vi "机械手工具坐标转世界坐标.vi"(9 "最终的世界坐标角度(单位角度)":dbl=89.996 format="%#_13g", 11 "P-XYZR":T2) -> (1 "计算出来 世界坐标系坐标XYZR out":T2, 3 "计算出来 世界坐标系坐标 out":T1 {"X" format="%#.3f"})   [LabVIEW 2014]
uses:
  Controls/XYPos.ctl
  Controls/XYZRPos.ctl
  Global.vi
panel:
  in  "选项卡控件":enum32{"选项卡 1", "选项卡 2"}(tab)=enum."选项卡 2"
  in  "世界坐标 O点(旧 R=0)":T1={"X"=309.781, "Y"=-196.165} {"X" format="%#.3f"}
  in  "OK工具坐标(robot显示)":T1={"X"=310.034, "Y"=-196.847} {"X" format="%#.3f"}
  out "OK offset":T1 {"X" format="%#.3f"}
  out "算出来 M在旧坐标系坐标":T1 {"X" format="%#.3f"}
  out "坐标平移量":cluster{dbl, dbl}
  in  "OK工具坐标 2":T1={"X"=309.781, "Y"=-194.165} {"X" format="%#.3f"}
  out "OK offset 2":T1 {"X" format="%#.3f"}
  out "算出来 M在旧坐标系坐标 2":T1 {"X" format="%#.3f"}
  out "计算的-坐标平移量 2":cluster{dbl, dbl}
  out "算出来 M在旧坐标系坐标 3":T1 {"X" format="%#.3f"}
  out "OK offset 3":T1 {"X" format="%#.3f"}
  in  "OK工具坐标(robot显示) 2":T1={"X"=310.033, "Y"=-196.846} {"X" format="%#.3f"}
  in  "工具/世界坐标XY in":T1={"X"=310.033, "Y"=-196.846} {"X" format="%#.3f"}
  in  "H0角度(单位角度)":dbl format="%#_13g"
  out "计算的-坐标平移量 3":cluster{dbl, dbl}
  in  "H0半径":dbl format="%#_13g"
  # "90"
  # "10"
  # "对位后世界坐标为XY  R\n求旋转后世界坐标\n1. XYR 转换为工具坐标 X1 Y1  R  (注意：这里仍然用世界坐标角度)\n2  H0旋转30度，则X1 Y1 (R+30)  \n3， 则X1 Y1 (R+30)  转换成世界坐标"
  # "309.352"
  # "-197.099"
  # "注意：这里输入的是最终世界坐标角度"
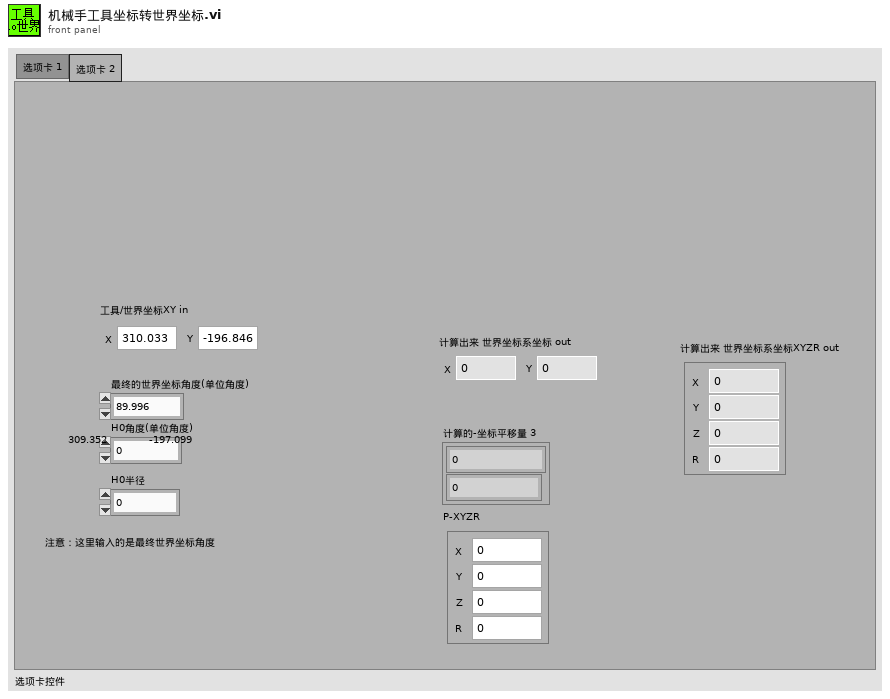
[diagram p1: front panel]
types:
  T1 = typedef "XYPos.ctl" = cluster{"X":dbl, "Y":dbl}
  T2 = typedef "XYZRPos.ctl" = cluster{"X":dbl, "Y":dbl, "Z":dbl, "R":dbl}
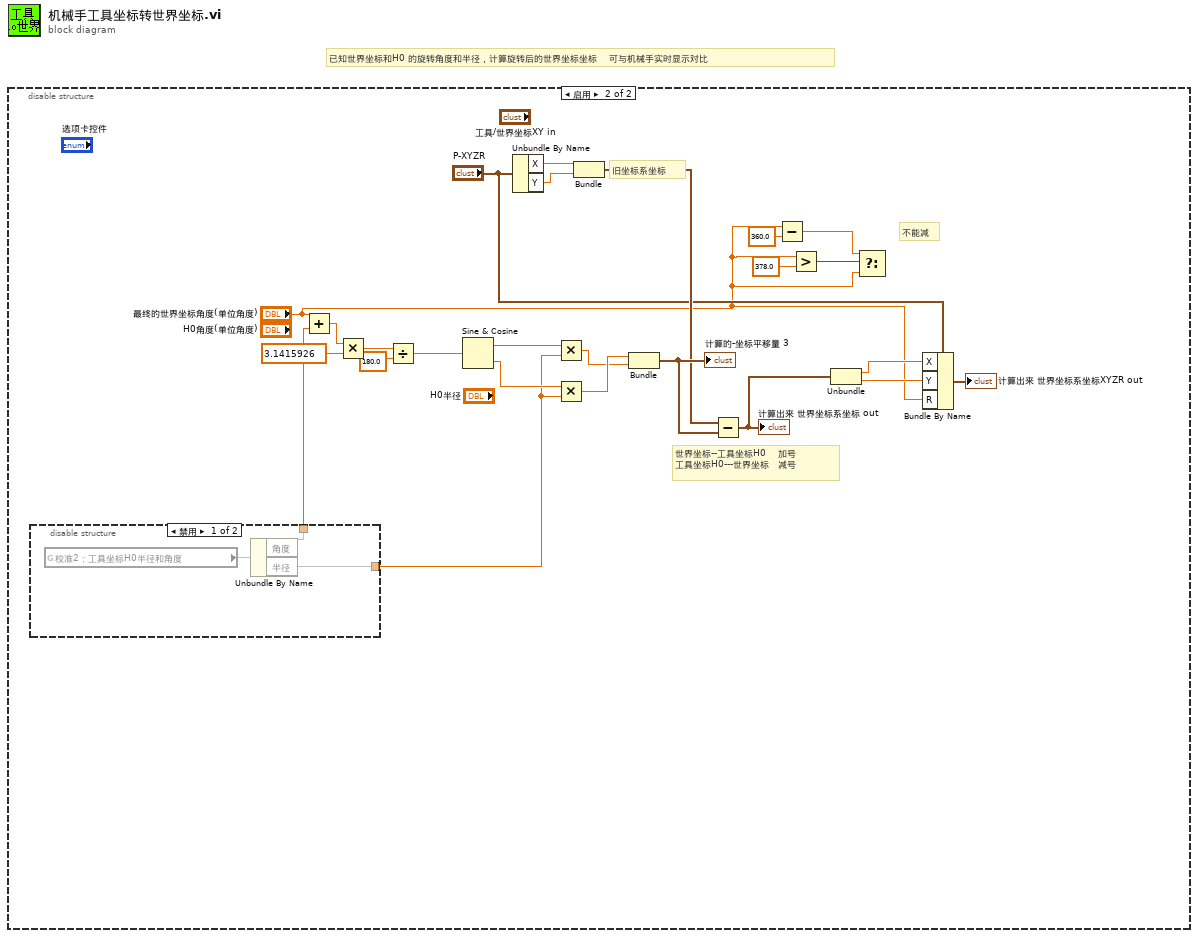
[diagram p0: block diagram]
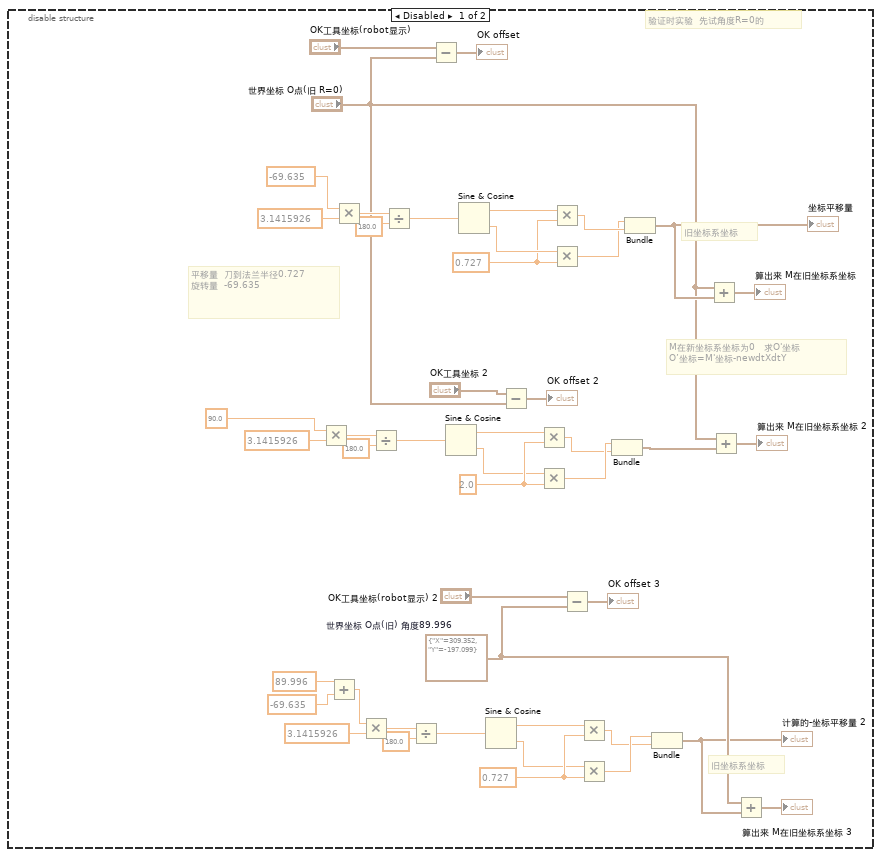
[diagram p2: hidden frame]
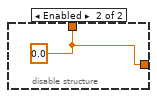
[diagram p3: hidden frame]
diagram:
  # "已知世界坐标和H0 的旋转角度和半径，计算旋转后的世界坐标坐标    可与机械手实时显示对比"
  n1 = disable-structure shown="启用" {
    frame Disabled {
      w17 = T1 {"X"=309.352, "Y"=-197.099}  # 世界坐标 O点(旧) 角度89.996
      w9 = 0.727 ("旋转角度(单位角度)")
      w26 = 2.0 ("旋转角度(单位角度)")
      w41 = 0.727 ("旋转角度(单位角度)")
      # "验证时实验  先试角度R=0的"
      # "旧坐标系坐标"
      # "旧坐标系坐标"
      # "M在新坐标系坐标为0   求O'坐标\nO’坐标=M'坐标-newdtXdtY"
      # "平移量  刀到法兰半径0.727\n旋转量  -69.635"
      n2 = Multiply(x=90.0 ("旋转角度(单位角度) 2"), y=3.1415926) -> (x*y=w22:dbl)
      n3 = Add(x=89.996 ("旋转角度(单位角度)"), y=-69.635 ("旋转角度(单位角度)")) -> (x+y=w1:dbl)
      n4 = Multiply(x=-69.635 ("旋转角度(单位角度)"), y=3.1415926) -> (x*y=w45:dbl)
      n5 = Multiply(x=w1, y=3.1415926) -> (x*y=w5:dbl)
      n6 = Divide(x=w22, y=180.0) -> (x/y=w30:dbl)
      n7 = Divide(x=w45, y=180.0) -> (x/y=w31:dbl)
      n8 = Divide(x=w5, y=180.0) -> (x/y=w16:dbl)
      n9 = Subtract(x="OK工具坐标(robot显示)", y="世界坐标 O点(旧 R=0)") -> (x-y=→"OK offset":T1)
      n10 = Sine & Cosine(0:w30) -> (1:w21:dbl, 2:w25:dbl)
      n11 = Sine & Cosine(0:w31) -> (1:w46:dbl, 2:w42:dbl)
      n12 = Sine & Cosine(0:w16) -> (1:w4:dbl, 2:w8:dbl)
      n13 = Subtract(x="OK工具坐标 2", y="世界坐标 O点(旧 R=0)") -> (x-y=→"OK offset 2":T1)
      n14 = Multiply(x=w21, y=w26) -> (x*y=w27:dbl)
      n15 = Multiply(x=w25, y=w26) -> (x*y=w28:dbl)
      n16 = Multiply(x=w46, y=w41) -> (x*y=w37:dbl)
      n17 = Multiply(x=w42, y=w41) -> (x*y=w36:dbl)
      n18 = Subtract(x="OK工具坐标(robot显示) 2", y=w17) -> (x-y=→"OK offset 3":T1)
      n19 = Multiply(x=w4, y=w9) -> (x*y=w13:dbl)
      n20 = Multiply(x=w8, y=w9) -> (x*y=w14:dbl)
      n21 = Bundle(w28, w27) -> (w18:cluster{dbl, dbl})  [unwired: 1 in]
      n22 = Bundle(w36, w37) -> (w38:cluster{dbl, dbl})  [unwired: 1 in]
      "坐标平移量" <- w38
      n23 = Bundle(w14, w13) -> (w12:cluster{dbl, dbl})  [unwired: 1 in]
      "计算的-坐标平移量 2" <- w12
      n24 = Add(x="世界坐标 O点(旧 R=0)", y=w38) -> (x+y=→"算出来 M在旧坐标系坐标":T1)
      n25 = Add(x="世界坐标 O点(旧 R=0)", y=w18) -> (x+y=→"算出来 M在旧坐标系坐标 2":T1)
      n26 = Add(x=w17, y=w12) -> (x+y=→"算出来 M在旧坐标系坐标 3":T1)
    }
    frame Enabled {
      # "不能减"
      # "世界坐标--工具坐标H0    加号\n工具坐标H0---世界坐标   减号"
      # "旧坐标系坐标"
      n27 = disable-structure shown="禁用" {
        disable-tunnel: [w73 w75] -> w53
        disable-tunnel: [w72 w75] -> w52
        frame Disabled {
          n28 = global read "Global.vi" "校准2：工具坐标H0半径和角度"() -> (w74)
          n29 = Unbundle By Name(w74) -> ("角度"=w72, "半径"=w73)
        }
        frame Enabled {
          w75 = 0.0
        }
      }
      n30 = Add(x="最终的世界坐标角度(单位角度)", y=w52) -> (x+y=w55:dbl)
      n31 = Multiply(x=w55, y=3.1415926) -> (x*y=w64:dbl)
      n32 = Divide(x=w64, y=180.0) -> (x/y=w71:dbl)
      n33 = Sine & Cosine(0:w71) -> (1:w63:dbl, 2:w67:dbl)
      n34 = Unbundle By Name("P-XYZR") -> ("X"=w62:dbl, "Y"=w61:dbl)
      n35 = Multiply(x=w63, y=w53) -> (x*y=w69:dbl)
      n36 = Multiply(x=w67, y=w53) -> (x*y=w70:dbl)
      n37 = Bundle("X"=w62, "Y"=w61) -> (w60:cluster{"X":dbl, "Y":dbl})  [unwired: 1 in]
      n38 = Bundle(w70, w69) -> (w68:cluster{dbl, dbl})  [unwired: 1 in]
      "计算的-坐标平移量 3" <- w68
      n39 = Subtract(x=w60, y=w68) -> (x-y=w59:cluster{dbl, dbl})
      "计算出来 世界坐标系坐标 out" <- w59
      n40 = Subtract(x="最终的世界坐标角度(单位角度)", y=360.0) -> (x-y=w48:dbl)
      n41 = Greater?(x="最终的世界坐标角度(单位角度)", y=378.0) -> (0:w50:bool)
      n42 = Unbundle(w59) -> (w57:dbl, w56:dbl)
      n43 = Select(t=w48, s=w50, f="最终的世界坐标角度(单位角度)") -> ()  [unwired: 1 out]
      n44 = Bundle By Name(cluster="P-XYZR", "X"=w57, "Y"=w56, "R"="最终的世界坐标角度(单位角度)") -> (→"计算出来 世界坐标系坐标XYZR out":T2)
    }
  }
